vi "task.vi"   [LabVIEW 2016, in "斯坦道总磷总氮.lvlib"]
types:
  T1 = typedef "控制命令与参数.ctl" = cluster{"控制命令":enum16{"启动测量", "标样核查", "零点核查", "跨度核查", "空白测试", "平行样测试", "加标回收", "空白校准", "标样校准", "初始化（清洗）", "停止测试", "仪器重启", "校时", "模式设置", "测量间隔设置"}, "测量参数":string}
  T2 = enum16{"启动测量", "标样核查", "零点核查", "跨度核查", "空白测试", "平行样测试", "加标回收", "空白校准", "标样校准", "初始化（清洗）", "停止测试", "仪器重启", "校时", "模式设置", "测量间隔设置"}
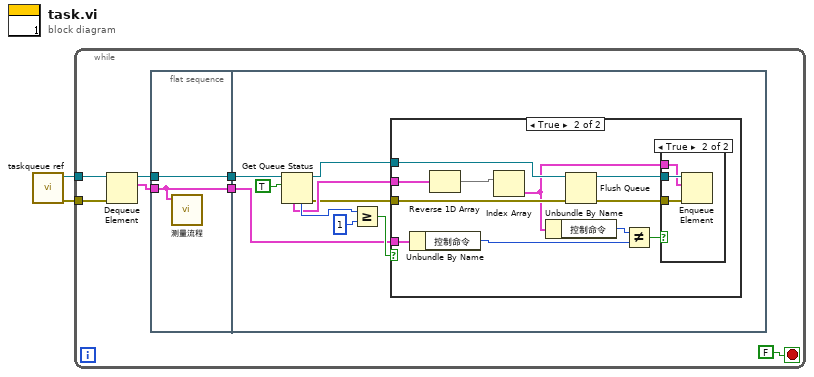
[diagram p0: block diagram]
diagram:
  n1 = call "taskqueue ref.vi"() -> ("错误输出"=w2:errorcluster, "队列输出"=w1:refnum<queue>)  [unwired: 10 in]
  n2 = while {
    tunnel: w1 -> [w8]
    tunnel: w2 -> [w6]
    stop <- FALSE stop-if-true
    n3 = Dequeue Element(queue=w8, error in (no error)=w6) -> (queue out=w5:refnum<queue>, element=w7:T1)  [unwired: 1 in, 2 out]
    n4 = flat-sequence {
      tunnel: w7 -> [w10]
      tunnel: w5 -> [w11]
      tunnel: [w11] -> w4
      tunnel: [w10] -> w3
      tunnel: w4 -> [w20]
      tunnel: w3 -> [w12]
      frame #0 {
        n5 = call "测量流程.vi"("输入参数"=w10) -> ()  [unwired: 11 in]
      }
      frame #1 {
        n6 = Get Queue Status(queue=w20, return elements? (F)=TRUE ("返回元素？(F)")) -> (queue out=w15:refnum<queue>, error out=w14:errorcluster, # elements in queue=w18:i32, elements=w16:T1[])  [unwired: 1 in, 4 out]
        n7 = Greater Or Equal?(x=w18, y=1) -> (x >= y?=w13:bool)
        n8 = case shown="True" w13 {
          tunnel: w16 -> [_ w31]
          tunnel: w15 -> [_ w29]
          tunnel: w14 -> [_ w28]
          tunnel: w12 -> [_ w25]
          frame False {
          }
          frame True {
            n9 = Unbundle By Name(w25) -> ("控制命令"=w23:T2)
            n10 = Reverse 1D Array(array=w31) -> (reversed array=w30:T1[])
            n11 = Index Array(array=w30) -> (element=w21:T1)  [unwired: 1 in]
            n12 = Unbundle By Name(w21) -> ("控制命令"=w24:T2)
            n13 = Flush Queue(queue=w29, error in (no error)=w28) -> (queue out=w27:refnum<queue>, error out=w26:errorcluster)  [unwired: 1 out]
            n14 = Not Equal?(x=w24, y=w23) -> (x != y?=w22:bool)
            n15 = case shown="True" w22 {
              tunnel: w27 -> [_ w34]
              tunnel: w26 -> [_ w33]
              tunnel: w21 -> [_ w32]
              frame False {
              }
              frame True {
                n16 = Enqueue Element(queue=w34, element=w32, error in (no error)=w33) -> ()  [unwired: 1 in, 3 out]
              }
            }
          }
        }
      }
    }
  }
